vi "I2C Write.vi"(7 "I2C Data Address Cluster":T2={"Data Address Endianness"=TRUE, " Data Address Width"=enum."2 Byte"}, 8 "error in (no error)":errorcluster, 9 "I2C Data Cluster":T1={"Address Byte"=0, "Number of Bytes"=0, "Page Size in Bytes"=128, "Data Byte"=[], "Write Delay Between Pages (ms)"=4} {"Data Byte" format="%02x"; "Address Byte" format="%04x"}, 10 "i2c configuration in":T4, 11 "device reference in":T3) -> (0 "error out":errorcluster, 1 "Data Bytes Written":u8[](array[numeric]) format="%02x", 2 "i2c configuration out":T4, 3 "device reference out":T3, 4 "I2C Data Cluster Out":T1={"Address Byte"=0, "Number of Bytes"=0, "Page Size in Bytes"=128, "Data Byte"=[], "Write Delay Between Pages (ms)"=4} {"Data Byte" format="%02x"; "Address Byte" format="%04x"})   [LabVIEW 2025]
doc: "This EEPROM example shows a more generalized way to use the I2C basic API to write data. It allows the user to change the following parameters: page size, write delay, the endianness of the address bytes, and the number of bytes in an address.\n\nThe parameters will have the following effects:\n\nTarget Page Size (bytes): This places an additional constraint on the amount of bytes written. The smaller value will be used, and that number of bytes written.\nWrite Delay Between Pages (ms): This will force a mandatory delay after writing bytes to a device.\nData Address Width: This will allow the user to specify the EEPROM Data Address as either 1 or 2 bytes.\nData Address Endianness: This control will change the ordering of the bytes in the EEPROM Data Address, note that this only has an effect if there are 2 bytes in the address.\n\nSince the I2C SDA and SCL lines are open-drain, they must be pulled up to the required reference voltage of your slave by connecting an appropriate resistor (2k-5k) between SCL and your reference voltage and SDA and your reference voltage. For NI-845x Hardware that contain internal pull-ups, you can use these. Otherwise, you need to use external pullups.\n\nFor connection information see the NI-845x Hardware and Software manual and the manual for your specific EEPROM."
uses:
  <vilib>/ni845x/ni845x.llb/ni845xI2cConfiguration.ctl
  <vilib>/ni845x/ni845x.llb/ni845xControl.ctl
  Type Definitions/I2C Data Address Cluster.ctl
  Type Definitions/I2C Data Cluster.ctl
panel:
  # "Big Endian"
  # "Little Endian"
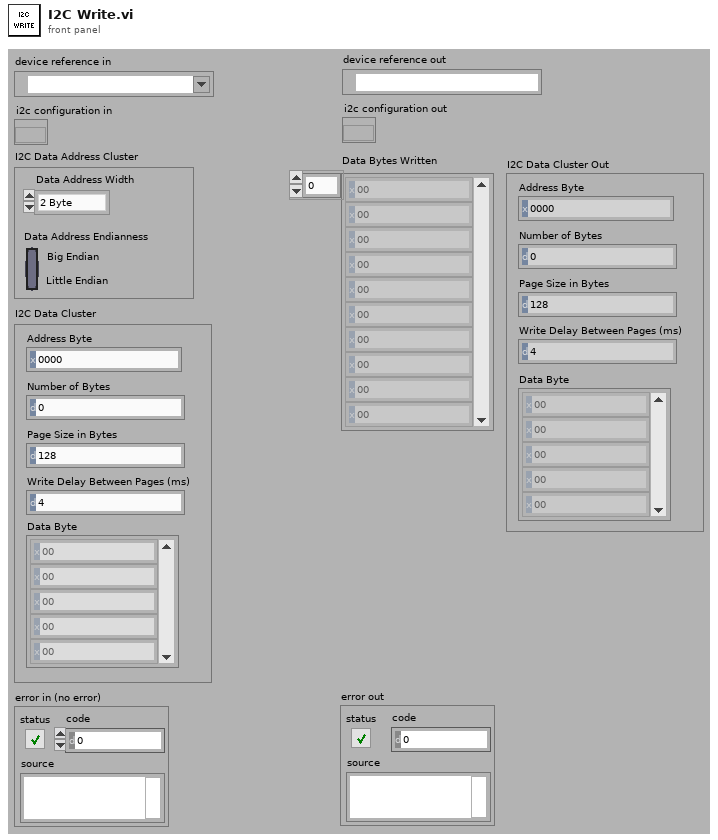
[diagram p1: front panel]
types:
  T1 = typedef "I2C Data Cluster.ctl" = cluster{"Address Byte":u16, "Number of Bytes":u32, "Page Size in Bytes":u32, "Data Byte":u8[], "Write Delay Between Pages (ms)":u32}
  T2 = typedef "I2C Data Address Cluster.ctl" = cluster{"Data Address Endianness":bool, " Data Address Width":enum16{"1 Byte", "2 Byte"}}
  T3 = typedef "ni845xControl.ctl" = refnum<k21>
  T4 = typedef "ni845xI2cConfiguration.ctl" = refnum<k20>
  T5 = cluster{"EEPROM Address":u16, "Length":u32, "Data Index":u32}[]
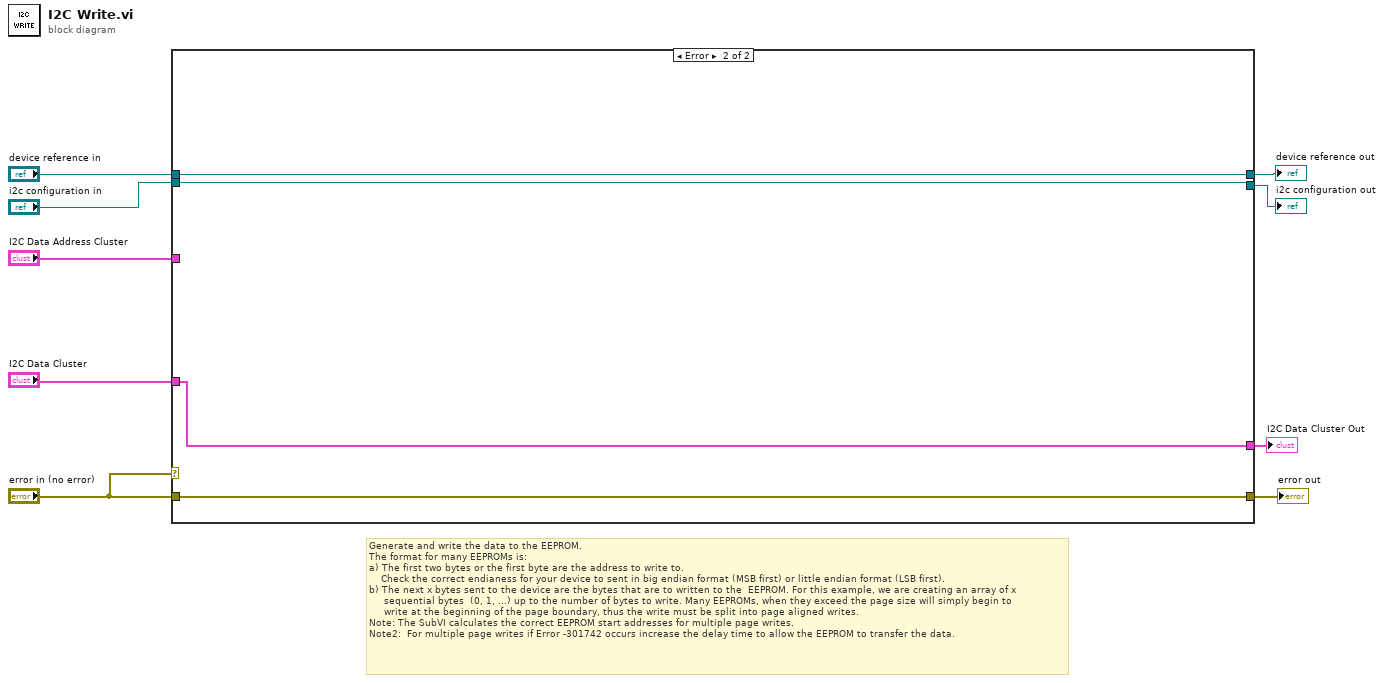
[diagram p0: block diagram]
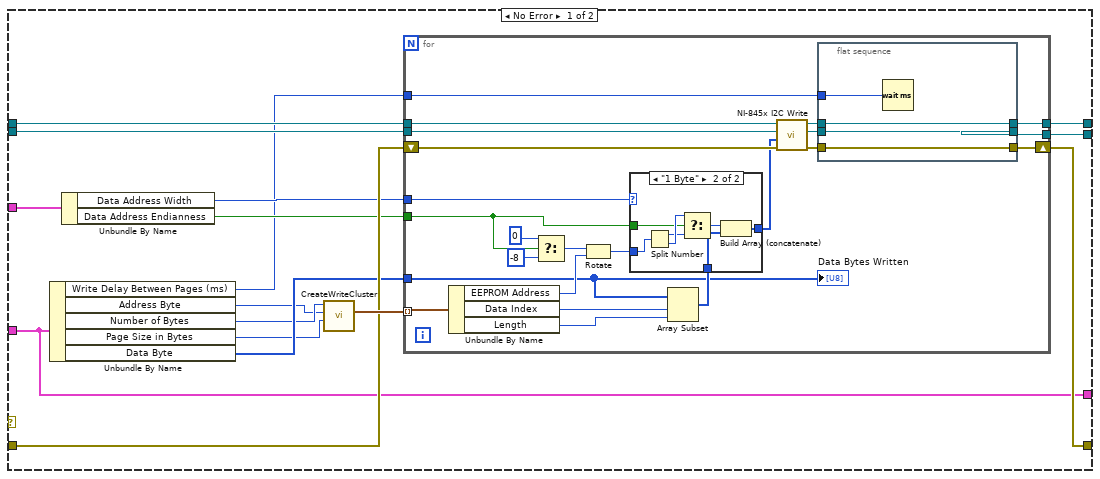
[diagram p2: hidden frame]
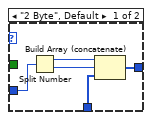
[diagram p3: hidden frame]
diagram:
  # "Generate and write the data to the EEPROM. \nThe format for many EEPROMs is:\na) The first two bytes or the first byte are the address to write to. \n    Check the correct endianess for your device to sent in big endian format (MSB first) or little endian format (LSB first).\nb) The next x bytes sent to the device are the bytes that are to written to the  EEPROM. For this example, we are creating an array of x\n     sequential bytes  (0, 1, ...) up to the number of bytes to write. Many EEPROMs, when they exceed the page size will simply begin to\n     write at the beginning of the page boundary, thus the write must be split into page aligned writes.\nNote: The SubVI calculates the correct EEPROM start addresses for multiple page writes.\nNote2:  For multiple page writes if Error -301742 occurs increase the delay time to allow the EEPROM to transfer the data."
  n1 = case shown="Error" "error in (no error)" {
    tunnel: "device reference in" -> [w24 w67]
    tunnel: "i2c configuration in" -> [w23 w66]
    tunnel: [w22 w67] -> w7
    tunnel: [w21 w66] -> w6
    tunnel: "error in (no error)" -> [w19 w68]
    tunnel: [w20 w68] -> w4
    tunnel: "I2C Data Cluster" -> [w10 w65]
    tunnel: "I2C Data Address Cluster" -> [w14 _]
    tunnel: [w10 w65] -> w1
    frame No Error {
      n2 = Unbundle By Name(w10) -> ("Write Delay Between Pages (ms)"=w11:u32, "Address Byte"=w16:u16, "Number of Bytes"=w17:u32, "Page Size in Bytes"=w15:u32, "Data Byte"=w18:u8[])
      n3 = Unbundle By Name(w14) -> ("Data Address Width"=w13:enum16{"1 Byte", "2 Byte"}, "Data Address Endianness"=w12:bool)
      n4 = call "CreateWriteCluster.vi"("Page Size in Bytes"=w15, "EEPROM Starting Address"=w16, "Number of Bytes to Write"=w17) -> ("Array of Write Cluster Information"=w25:T5)  [unwired: 1 out]
      n5 = for {
        shift-right: [w48] -> w20
        shift-left: w19 -> [w45]
        tunnel: w18 -> [w28]
        tunnel: w24 -> [w43]
        tunnel: [w47] -> w22
        tunnel: w23 -> [w46]
        tunnel: [w35] -> w21
        tunnel: w25 -> [w30] mode=indexing
        tunnel: w13 -> [w29]
        tunnel: w12 -> [w26]
        tunnel: w11 -> [w27]
        n6 = Unbundle By Name(w30) -> ("EEPROM Address"=w31:u16, "Data Index"=w32:u32, "Length"=w33:u32)
        n7 = Select(t=i16 0, s=w26, f=i16 -8) -> (s? t:f=w39:i16)
        n8 = Rotate(1:w31, 2:w39) -> (0:w38:u16)
        n9 = Array Subset(array=w28, index=w32, length=w33) -> (w34:u8[])
        n10 = case shown="\"1 Byte\"" w29 {
          tunnel: w38 -> [w53 w58]
          tunnel: [w52 w60] -> w37
          tunnel: w34 -> [w51 w59]
          tunnel: w26 -> [_ w54]
          frame "2 Byte", Default {
            n11 = Split Number(x=w53) -> (hi(x)=w49:u8, lo(x)=w50:u8)
            n12 = Build Array (concatenate)(w49, w50, w51) -> (w52:u8[])
          }
          frame "1 Byte" {
            n13 = Split Number(x=w58) -> (hi(x)=w55:u8, lo(x)=w56:u8)
            n14 = Select(t=w56, s=w54, f=w55) -> (s? t:f=w57:u8)
            n15 = Build Array (concatenate)(w57, w59) -> (w60:u8[])
          }
        }
        n16 = call <vilib>:"NI-845x I2C Write.vi"("error in (no error)"=w45, "write data"=w37, "i2c configuration in"=w46, "device reference in"=w43) -> ("error out"=w44:errorcluster, "i2c configuration out"=w36:T4, "device reference out"=w42:T3)  [unwired: 5 out]
        n17 = flat-sequence {
          tunnel: [w64] -> w48
          tunnel: [w63] -> w47
          tunnel: w42 -> [w63]
          tunnel: w44 -> [w64]
          tunnel: w36 -> [w62]
          tunnel: [w62] -> w35
          tunnel: w27 -> [w61]
          frame #0 {
            n18 = Wait (ms)(milliseconds to wait=w61) -> ()  [unwired: 1 out]
          }
        }
        "Data Bytes Written" <- w28
      }
    }
    frame Error {
    }
  }
  "i2c configuration out" <- w6
  "device reference out" <- w7
  "error out" <- w4
  "I2C Data Cluster Out" <- w1
